vi "Trapezoid Profile.vi"(6 "Limits":T1, 8 "dt":dbl, 11 "goal":dbl) -> (0 "x_rec":dbl[](array[numeric]), 3 "v_rec":dbl[](array[numeric]), 4 "t_rec":dbl[](array[numeric]))   [LabVIEW 2025]
panel:
  out "a_rec":dbl[](array[numeric])
  out "Velocity Graph":cluster{"v_rec":dbl[], "a_rec":dbl[]}[](graph)
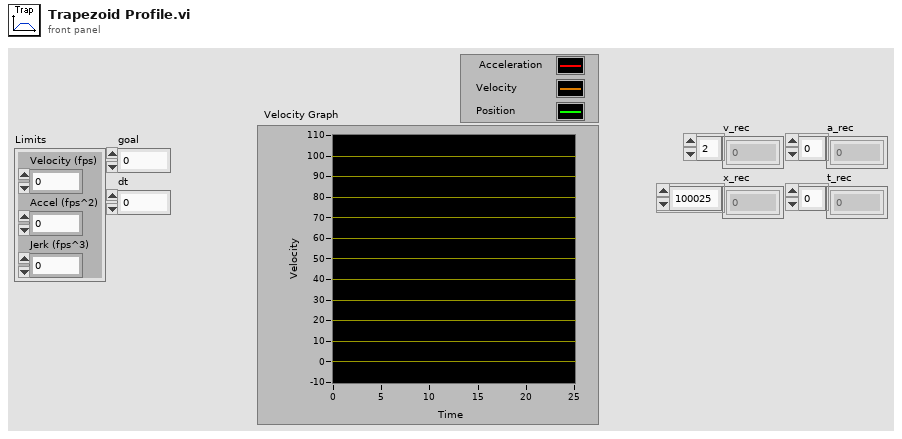
[diagram p1: front panel]
types:
  T1 = cluster{"Velocity (fps)":dbl, "Accel (fps^2)":dbl, "Jerk (fps^3)":dbl}
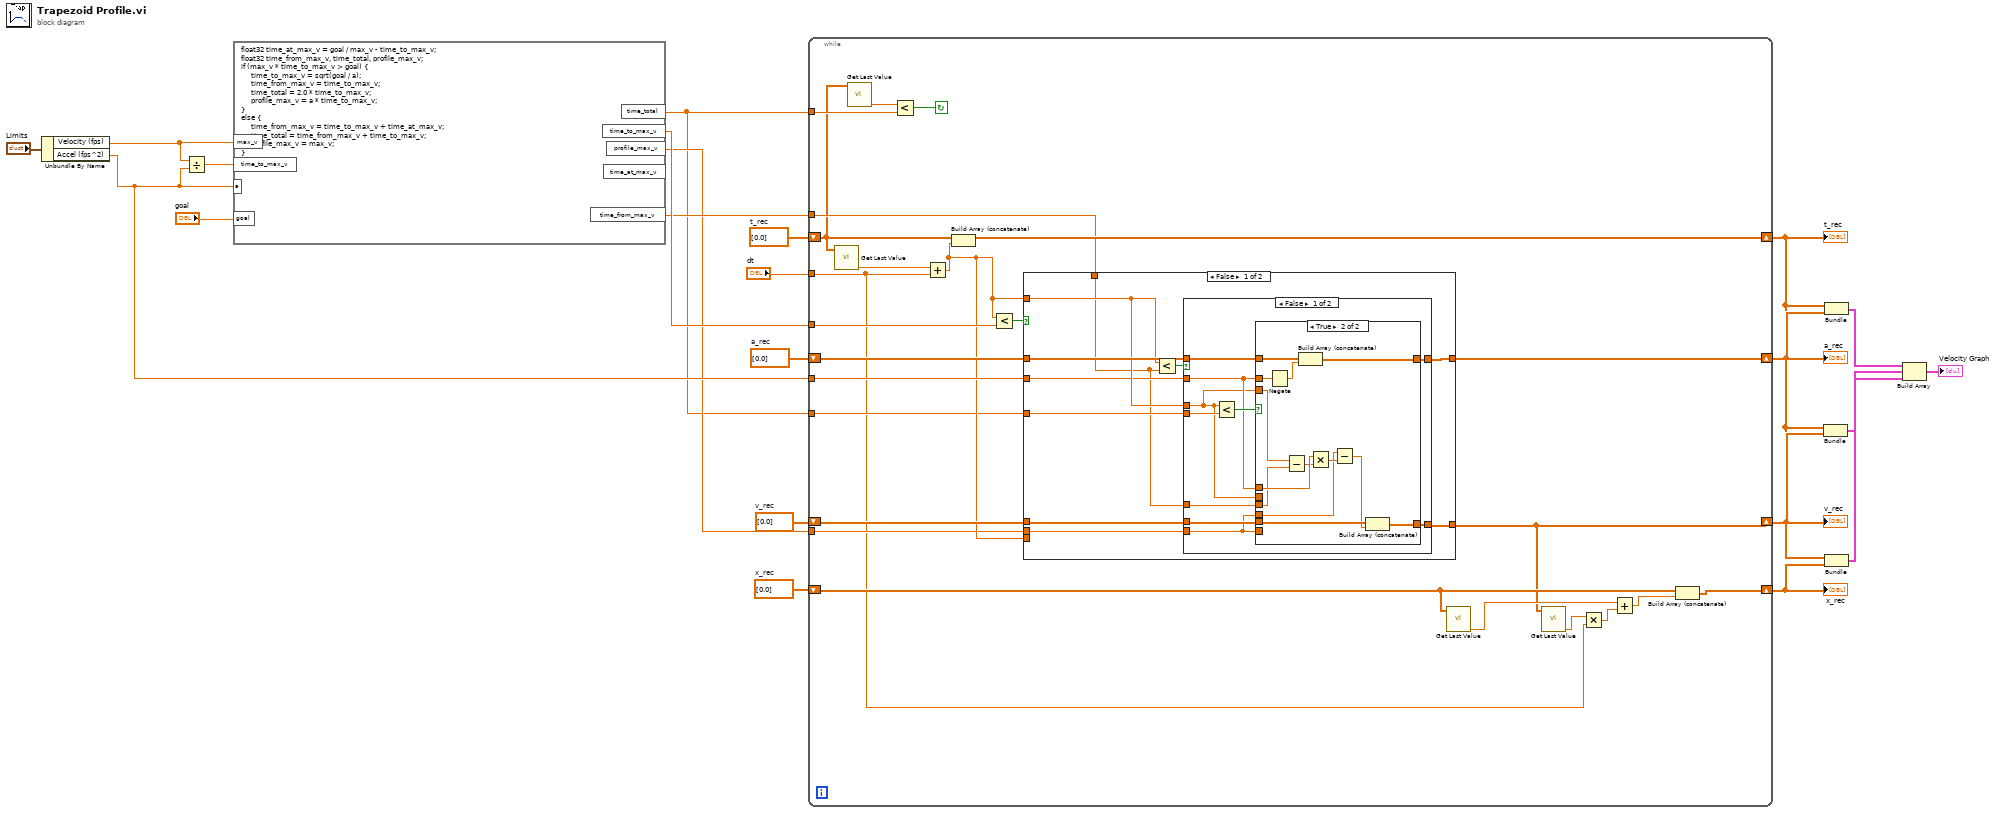
[diagram p0: block diagram]
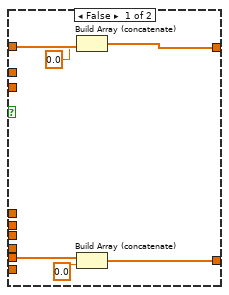
[diagram p2: hidden frame]
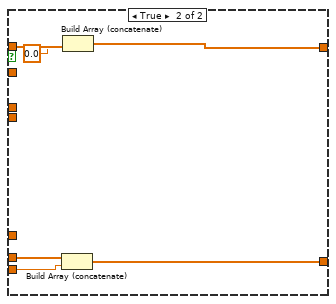
[diagram p3: hidden frame]
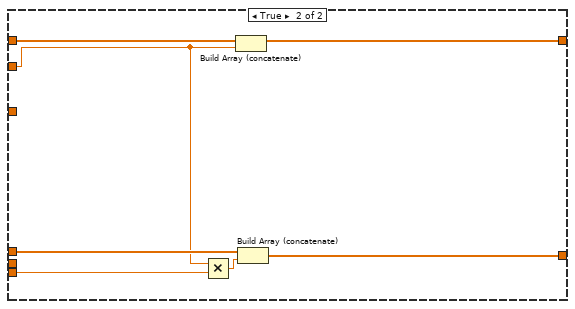
[diagram p4: hidden frame]
diagram:
  w1 = dbl[] [0.0]  # v_rec
  w13 = dbl[] [0.0]  # x_rec
  w14 = dbl[] [0.0]  # a_rec
  w15 = dbl[] [0.0]  # t_rec
  n1 = Unbundle By Name("Limits") -> ("Velocity (fps)"=w2:dbl, "Accel (fps^2)"=w17:dbl)
  n2 = Divide(x=w2, y=w17) -> (x/y=w21:dbl)
  n3 = formula code="float32 time_at_max_v = goal / max_v - time_to_max_v;\nfloat32 time_from_max_v, time_total, profile_max_v;\nif (max_v * time_to_max_v > goal) {\n     time_to_max_v = sqrt(goal / a);\n     time_from_max_v = time_to_max_v;\n     time_total = 2.0 * time_to_max_v;\n     profile_max_v = a * time_to_max_v;\n}\nelse {\n     time_from_max_v = time_to_max_v + time_at_max_v;\n     time_total = time_from_max_v + time_to_max_v;\n     profile_max_v = max_v;\n}"("max_v"=w2, "time_to_max_v"=w21, "goal"="goal", "a"=w17) -> ("time_to_max_v"=w18:dbl, "profile_max_v"=w12:sgl, "time_total"=w11:sgl, "time_from_max_v"=w16:sgl)  [unwired: 1 out]
  n4 = while {
    shift-right: [w33] -> w5
    shift-left: w13 -> [w28]
    shift-right: [w27] -> w6
    shift-left: w1 -> [w38]
    shift-right: [w39] -> w10
    shift-left: w14 -> [w41]
    shift-right: [w44] -> w4
    shift-left: w15 -> [w31]
    tunnel: w11 -> [w45]
    tunnel: "dt" -> [w24]
    tunnel: w18 -> [w42]
    tunnel: w17 -> [w40]
    tunnel: w16 -> [w36]
    tunnel: w12 -> [w35]
    tunnel: w11 -> [w34]
    stop <- w46 continue-if-true
    n5 = call "Get Last Value.vi"("array"=w31) -> ("element"=w30:dbl)  [unwired: 10 in]
    n6 = call "Get Last Value.vi"("array"=w31) -> ("element"=w32:dbl)  [unwired: 10 in]
    n7 = Less?(x=w32, y=w45) -> (x < y?=w46:bool)
    n8 = Add(x=w30, y=w24) -> (x+y=w37:dbl)
    n9 = Build Array (concatenate)(w31, w37) -> (w44:dbl[])
    n10 = Less?(x=w37, y=w42) -> (x < y?=w43:bool)
    n11 = case shown="False" w43 {
      tunnel: w41 -> [w55 w98]
      tunnel: w40 -> [w48 w93]
      tunnel: [w54 w97] -> w39
      tunnel: w38 -> [w53 w96]
      tunnel: w37 -> [_ w94]
      tunnel: [w51 w92] -> w27
      tunnel: w37 -> [w49 _]
      tunnel: w36 -> [w47 _]
      tunnel: w35 -> [w52 _]
      tunnel: w34 -> [w50 _]
      frame False {
        n12 = Less?(x=w49, y=w47) -> (x < y?=w56:bool)
        n13 = case shown="False" w56 {
          tunnel: w55 -> [w64 w91]
          tunnel: [w63 w89] -> w54
          tunnel: w53 -> [w62 w88]
          tunnel: w52 -> [w58 w87]
          tunnel: [w61 w86] -> w51
          tunnel: w50 -> [w66 _]
          tunnel: w49 -> [w57 _]
          tunnel: w48 -> [w59 _]
          tunnel: w47 -> [w60 _]
          frame False {
            n14 = Less?(x=w57, y=w66) -> (x < y?=w65:bool)
            n15 = case shown="True" w65 {
              tunnel: w64 -> [w72 w85]
              tunnel: w59 -> [_ w80]
              tunnel: [w71 w83] -> w63
              tunnel: w62 -> [w68 w82]
              tunnel: w58 -> [_ _]
              tunnel: [w67 w81] -> w61
              tunnel: w57 -> [_ _]
              tunnel: w60 -> [_ w73]
              tunnel: w59 -> [_ w77]
              tunnel: w58 -> [_ w76]
              tunnel: w57 -> [_ w74]
              frame False {
                n16 = Build Array (concatenate)(w72, 0.0) -> (w71:dbl[])
                n17 = Build Array (concatenate)(w68, 0.0) -> (w67:dbl[])
              }
              frame True {
                n18 = Negate(x=w80) -> (-x=w84:dbl)
                n19 = Subtract(x=w74, y=w73) -> (x-y=w75:dbl)
                n20 = Build Array (concatenate)(w85, w84) -> (w83:dbl[])
                n21 = Multiply(x=w77, y=w75) -> (x*y=w79:dbl)
                n22 = Subtract(x=w76, y=w79) -> (x-y=w78:dbl)
                n23 = Build Array (concatenate)(w82, w78) -> (w81:dbl[])
              }
            }
          }
          frame True {
            n24 = Build Array (concatenate)(w88, w87) -> (w86:dbl[])
            n25 = Build Array (concatenate)(w91, 0.0) -> (w89:dbl[])
          }
        }
      }
      frame True {
        n26 = Multiply(x=w93, y=w94) -> (x*y=w95:dbl)
        n27 = Build Array (concatenate)(w98, w93) -> (w97:dbl[])
        n28 = Build Array (concatenate)(w96, w95) -> (w92:dbl[])
      }
    }
    n29 = call "Get Last Value.vi"("array"=w28) -> ("element"=w29:dbl)  [unwired: 10 in]
    n30 = call "Get Last Value.vi"("array"=w27) -> ("element"=w26:dbl)  [unwired: 10 in]
    n31 = Multiply(x=w26, y=w24) -> (x*y=w25:dbl)
    n32 = Add(x=w29, y=w25) -> (x+y=w23:dbl)
    n33 = Build Array (concatenate)(w28, w23) -> (w33:dbl[])
  }
  "v_rec" <- w6
  "x_rec" <- w5
  "a_rec" <- w10
  "t_rec" <- w4
  n34 = Bundle("t_rec"=w4, "v_rec"=w6) -> (w9:cluster{"t_rec":dbl[], "v_rec":dbl[]})  [unwired: 1 in]
  n35 = Bundle("t_rec"=w4, "a_rec"=w10) -> (w8:cluster{"t_rec":dbl[], "a_rec":dbl[]})  [unwired: 1 in]
  n36 = Bundle("t_rec"=w4, "x_rec"=w5) -> (w3:cluster{"t_rec":dbl[], "x_rec":dbl[]})  [unwired: 1 in]
  n37 = Build Array(w8, w9, w3) -> (→"Velocity Graph":cluster{"t_rec":dbl[], "x_rec":dbl[]}[])
